vi "DSC_Create Process.vi"   [LabVIEW 2013]
uses:
  <vilib>/lvdsc/NI_DSC.lvlib
types:
  T1 = cluster{"machine":string, "name":string, "path":path}
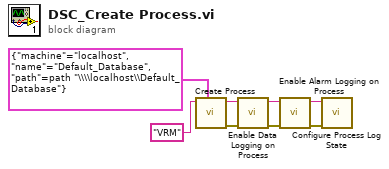
[diagram p0: block diagram]
diagram:
  n1 = call <vilib>:"Create Process.vi"("data database"=T1 {"machine"="localhost", "name"="Default_Database", "path"=path "\\\\localhost\\Default_Database"}, "process name"="VRM") -> ("error out"=w5:errorcluster, "process name out"=w6:string)  [unwired: 8 in]
  n2 = call <vilib>:"Enable Data Logging on Process.vi"("error in (no error)"=w5, "process name"=w6) -> ("error out"=w4:errorcluster, "process name out"=w3:string)  [unwired: 8 in]
  n3 = call <vilib>:"Enable Alarm Logging on Process.vi"("error in (no error)"=w4, "process name"=w3) -> ("error out"=w2:errorcluster, "process name out"=w1:string)  [unwired: 8 in]
  n4 = call <vilib>:"Configure Process Log State.vi"("error in (no error)"=w2, "process name"=w1) -> ()  [unwired: 8 in, 2 out]
